vi "数据拟合.vi"(8 "polynomial order":i32=2 caption="多项式阶数", 9 "拟合方法":u16(ring) items=["最小二乘", "最小绝对残差", "Bisquare"], 10 "Y":dbl[](array[numeric]), 11 "X":dbl[](array[numeric])) -> (1 "XY图":cluster{"X Values":dbl[], "Y Values":dbl[]}[](graph), 2 "拟合方程":string, 3 "拟合数据":dbl[](array[numeric]) format="%#.6g")   [LabVIEW 2021]
uses:
  <vilib>/Analysis/NI_AALPro.lvlib
  <vilib>/gmath/NI_Gmath.lvlib
panel:
  out "均方差":dbl format="%#.3g"
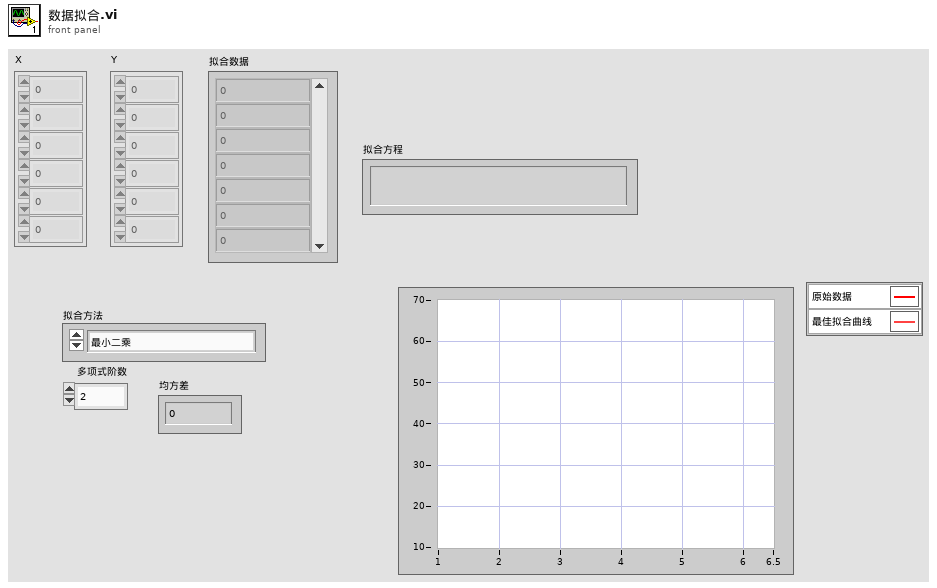
[diagram p1: front panel]
types:
  T1 = enum16{"Linear", "Polynomial", "Exponential", "Power"}
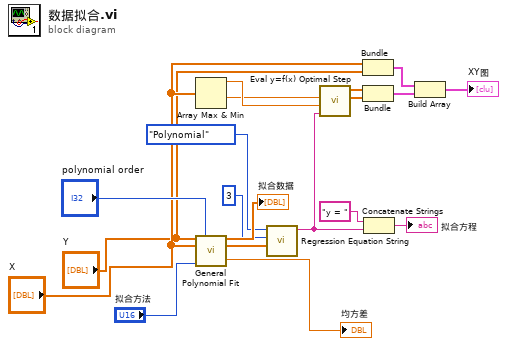
[diagram p0: block diagram]
diagram:
  n1 = Array Max & Min(array="X") -> (max value=w10:dbl, min value=w6:dbl)  [unwired: 2 out]
  n2 = call <vilib>:"General Polynomial Fit.vi"("Y"="Y", "polynomial order"="polynomial order", "X"="X", "method"="拟合方法") -> ("Best Polynomial Fit"=→"拟合数据":dbl[], "Polynomial Coefficients"=w17:dbl[], "residue"=→"均方差":dbl)  [unwired: 8 in, 1 out]
  n3 = call "Regression Equation String.vi"("系数"=w17, "精度"=3, "拟合类型"=T1."Polynomial" ("fit type")) -> ("公式"=w7:string)  [unwired: 8 in]
  n4 = call <vilib>:"Eval y=f(x) Optimal Step.vi"("formula"=w7, "end"=w10, "start"=w6) -> ("Y Values"=w12:dbl[], "X Values"=w13:dbl[])  [unwired: 2 in, 2 out]
  n5 = Bundle("X"="X", "Y"="Y") -> (w18:cluster{"X":dbl[], "Y":dbl[]})  [unwired: 1 in]
  n6 = Bundle("X Values"=w13, "Y Values"=w12) -> (w15:cluster{"X Values":dbl[], "Y Values":dbl[]})  [unwired: 1 in]
  n7 = Concatenate Strings("y = " ("string"), w7) -> (→"拟合方程":string)
  n8 = Build Array(w18, w15) -> (→"XY图":cluster{"X Values":dbl[], "Y Values":dbl[]}[])
